vi "Constants.vi"() -> ()   [LabVIEW 2017, in "Exercise 7.2 Shared.lvlib"]
doc: "Use this Global VI to access the GUIDs assigned to the page resources of the Custom Device."
uses:
  Exercise 7.2 Shared.lvlib
panel:
  in  "Tab Control":enum32{"GUIDS", "Constants", "Properties"}(tab)
  in  "Exercise 7.2":string="a6412327-4537-4c33-a507-80c95b83f1fc"
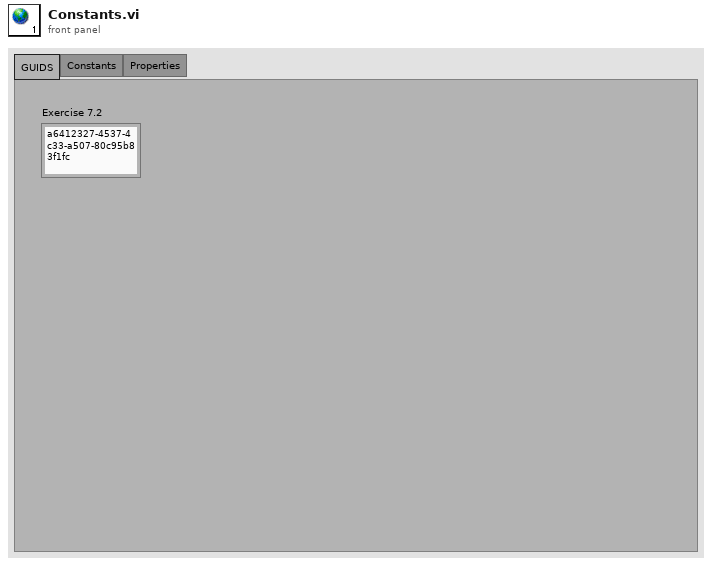
[diagram p1: front panel]
diagram:
